vi "aft_Get_AFT_Filter_Type_Sub.vi"(10 "adaptive filter in":refnum<k20>) -> (0 "error":i32, 3 "type":i32(ring) items=["LMS Real", "LMS Complex", "Normalized LMS Real", "Normalized LMS Complex", "Filtered-X LMS", "Normalized Filtered-X LMS", "Sign LMS", "Fast Block LMS", "RLS Real", "RLS Complex", "QR decomposition RLS Real", "QR decomposition RLS Complex"])   [LabVIEW 2017, in "NI_AdaptiveFilter.lvlib"]
doc: "Get adaptive filter type."
uses:
  <vilib>/addons/Adaptive Filters/NI_AdaptiveFilter.lvlib
  <resource>/AdaptiveFilters.dll
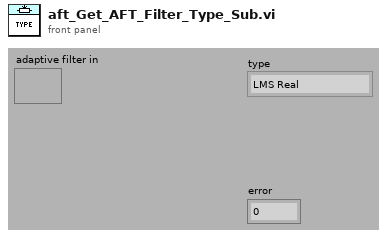
[diagram p1: front panel]
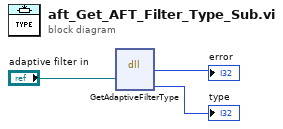
[diagram p0: block diagram]
diagram:
  n1 = dll-call lib="C:/Program Files/National Instruments/LabVIEW 2017/resource/AdaptiveFilters.dll" fn="GetAdaptiveFilterType" ("Complex Data Initialization")("pSession"="adaptive filter in") -> ("err"=→"error":i32, "type"=→"type":i32)  [unwired: 4 in, 3 out]
